vi "readFromSpreadsheetToArrays.vi"(11 "file path (dialog if empty)":path) -> (0 "column4":dbl[](array[numeric]), 1 "column3":dbl[](array[numeric]), 2 "column2":dbl[](array[numeric]), 3 "column1":dbl[](array[numeric]))   [LabVIEW 2015]
uses:
  <vilib>/Utility/file.llb/Read Delimited Spreadsheet (DBL).vi
panel:
  out "all rows":dbl[][](array[numeric])
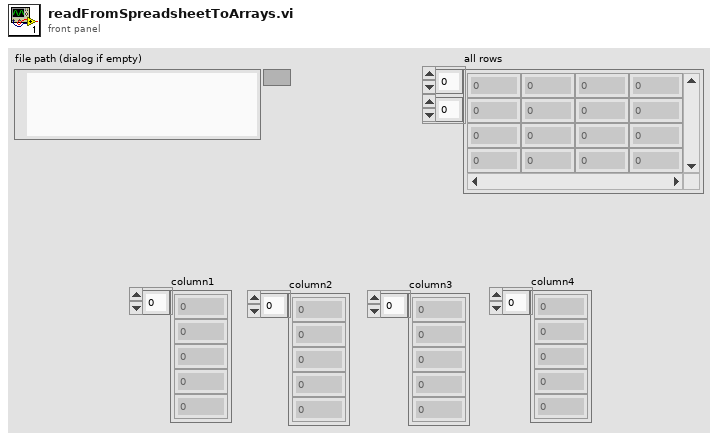
[diagram p1: front panel]
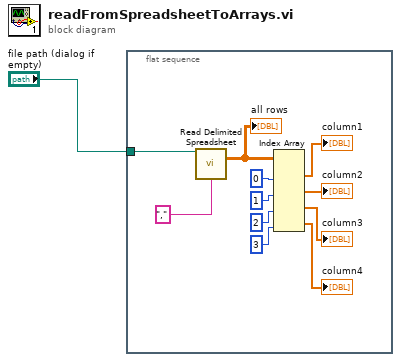
[diagram p0: block diagram]
diagram:
  n1 = flat-sequence {
    tunnel: "file path (dialog if empty)" -> [w2]
    frame #0 {
      n2 = call-poly <vilib>:"Read Delimited Spreadsheet.vi"("file path (dialog if empty)"=w2, "delimiter (\\t)"="," ("delimiter (\\t)")) -> ("all rows"=w4:dbl[][])  [unwired: 8 in, 5 out]
      "all rows" <- w4
      n3 = Index Array(array=w4, index (col) #1=0 ("disabled index (col)"), index (col) #2=1 ("index (col)"), index (col) #3=2 ("index (col)"), index (col) #4=3 ("index (col)")) -> (element #1=→"column1":dbl[], element #2=→"column2":dbl[], element #3=→"column3":dbl[], element #4=→"column4":dbl[])  [unwired: 4 in]
    }
  }
